vi "Do Cleaning Service.vi"(10 "Action":T1, 11 "Hotel":string) -> ()   [LabVIEW 2023]
doc: "This VI starts or stops the cleaning service for the given hotel."
uses:
  Do Cleaning Action.ctl
  <vilib>/Utility/miscctls.llb/LVRectTypeDef.ctl
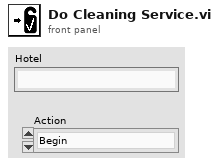
[diagram p1: front panel]
types:
  T1 = typedef "Do Cleaning Action.ctl" = enum16{"Begin", "End"}
  T2 = enum32{"Invalid", "Standard", "Closed", "Hidden", "Minimized", "Maximized"}
  T3 = typedef "LVRectTypeDef.ctl" = cluster{"Left":i16, "Top":i16, "Right":i16, "Bottom":i16}
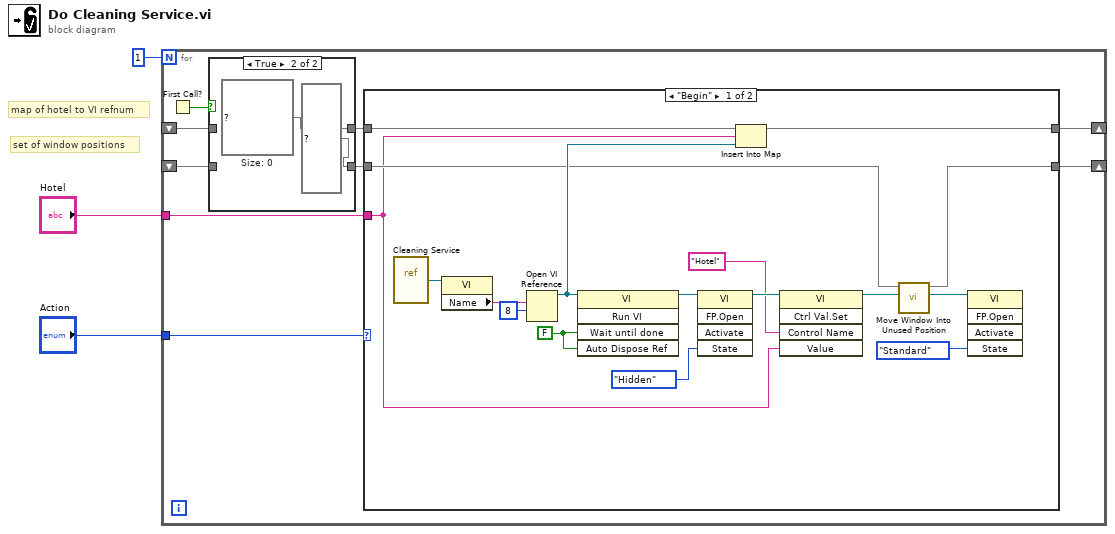
[diagram p0: block diagram]
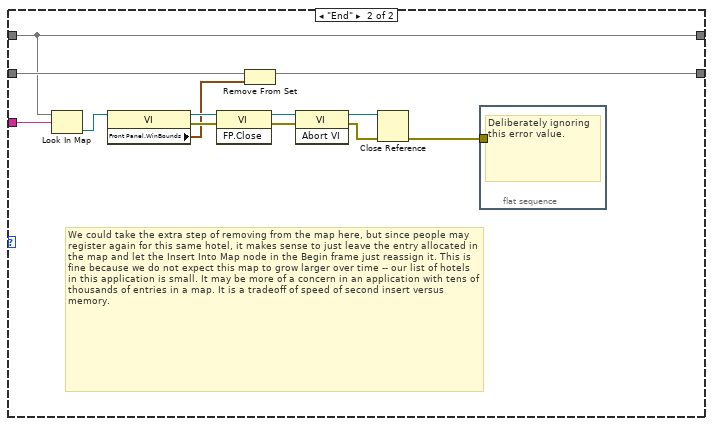
[diagram p2: hidden frame]
diagram:
  # "set of window positions"
  # "map of hotel to VI refnum"
  n1 = for {
    N: 1 -> [_]
    shift-right: [w4] -> _
    shift-left: _ -> [w11]
    tunnel: "Hotel" -> [w9]
    tunnel: "Action" -> [w8]
    shift-right: [w5] -> _
    shift-left: _ -> [w7]
    n2 = First Call?() -> (First Call?: T/F=w12:bool)
    n3 = case shown="True" w12 {
      tunnel: w11 -> [w44 _]
      tunnel: [w44 w46] -> w10
      tunnel: w7 -> [w43 _]
      tunnel: [w43 set{T3} {} ("set out")] -> w6
      frame False {
      }
      frame True {
        w46 = map{string, refnum<vi>} {}  # Size: 0
      }
    }
    n4 = case shown="\"Begin\"" w8 {
      tunnel: w10 -> [w29 w32]
      tunnel: w9 -> [w16 w31]
      tunnel: [w28 w32] -> w4
      tunnel: w6 -> [w20 w35]
      tunnel: [w21 w34] -> w5
      frame "Begin" {
        w23 = FALSE ("Wait Until Done")
        n5 = vi-ref "Cleaning Service.vi"() -> (w27:refnum<vi>)
        n6 = property class="VI"(reference=w27) -> ("Name"=w26:string)  [unwired: 1 in, 2 out]
        n7 = Open VI Reference(vi path=w26, options=8) -> (vi reference=w24:refnum<vi>)  [unwired: 4 in, 1 out]
        n8 = invoke class="VI" method="Run VI"(reference=w24, "Wait until done"=w23, "Auto Dispose Ref"=w23) -> (reference out=w22:refnum<vi>)  [unwired: 2 in, 4 out]
        n9 = invoke class="VI" method="FP.Open"(reference=w22, "State"=T2."Hidden") -> (reference out=w19:refnum<vi>)  [unwired: 3 in, 4 out]
        n10 = Insert Into Map(map in=w29, key=w16, value=w24) -> (map out=w28:map{string, refnum<vi>})  [unwired: 2 out]
        n11 = invoke class="VI" method="Ctrl Val.Set"(reference=w19, "Control Name"="Hotel" ("L10n_control name"), "Value"=w16) -> (reference out=w18:refnum<vi>)  [unwired: 2 in, 4 out]
        n12 = call "Move Window Into Unused Position.vi"("VI in"=w18, "set in"=w20) -> ("VI out"=w14:refnum<vi>, "set out"=w21:set{T3})  [unwired: 8 in]
        n13 = invoke class="VI" method="FP.Open"(reference=w14, "State"=T2."Standard") -> ()  [unwired: 3 in, 5 out]
      }
      frame "End" {
        # "We could take the extra step of removing from the map here, but since people may register again for this same hotel, it makes sense to just leave the entry allocated in the map and let the Insert Into Map node in the Begin frame just reassign it. This is fine because we do not expect this map to grow larger over time -- our list of hotels in this application is small. It may be more of a concern in an application with tens of thousands of entries in a map. It is a tradeoff of speed of second insert versus memory."
        n14 = Look In Map(map=w32, key=w31) -> (value=w30:refnum<vi>)  [unwired: 1 in, 1 out]
        n15 = property class="VI"(reference=w30) -> (reference out=w37:refnum<vi>, error out=w36:errorcluster, "Front Panel.WinBounds"=w33:T3)  [unwired: 1 in]
        n16 = invoke class="VI" method="FP.Close"(reference=w37, error in=w36) -> (reference out=w42:refnum<vi>, error out=w40:errorcluster)  [unwired: 1 in, 1 out]
        n17 = Remove From Set(10:w33, 11:w35) -> (3:w34:set{T3})  [unwired: 1 out]
        n18 = invoke class="VI" method="Abort VI"(reference=w42, error in=w40) -> (reference out=w41:refnum<vi>, error out=w39:errorcluster)  [unwired: 1 in, 1 out]
        n19 = Close Reference(reference=w41, error in (no error)=w39) -> (error out=w38:errorcluster)
        n20 = flat-sequence {
          tunnel: w38 -> [_]
          frame #0 {
            # "Deliberately ignoring this error value."
          }
        }
      }
    }
  }
